vi "Initialize.vi"(7 "Serial Configuration":T1={"Baud Rate"=57600, "Parity"=1, "Data Bits"=7, "Stop Bits"=10, "Flow Control"=0} {"Flow Control" items=["None", "XON/XOFF", "RTS/CTS", "XON/XOFF & RTS/CTS", "DTR/DSR", "XON/XOFF & DTR/DSR"]; "Stop Bits" items=["1.0"=10, "1.5"=15, "2.0"=20]; "Data Bits" items=["7"=7, "8"=8]; "Parity" items=["None", "Odd", "Even", "Mark", "Space"]; "Baud Rate" items=["300"=300, "600"=600, "1200"=1200, "2400"=2400, "4800"=4800, "9600"=9600, "19200"=19200, "38400"=38400, "57600"=57600]}, 8 "error in (no error)":errorcluster, 9 "Reset (True)":bool=TRUE, 10 "ID Query (True)":bool=TRUE, 11 "VISA resource name":refnum<visa-resource-name>) -> (0 "error out":errorcluster, 3 "VISA resource name out":refnum<visa-resource-name>)   [LabVIEW 2015, in "Lake Shore 350.lvlib"]
doc: "Establishes communication with the instrument and optionally performs an instrument identification query and/or an instrument reset. It also places the instrument in a default state needed for other instrument driver operations. Therefore, call this VI before calling other instrument driver VIs for this instrument. Generally, you need to call the <B>Initialize VI</B> only once at the beginning of an application."
uses:
  Lake Shore 350.lvlib
panel:
  # "(c) 2013 Lake Shore Cryotronics Inc.  ALL RIGHTS RESERVED."
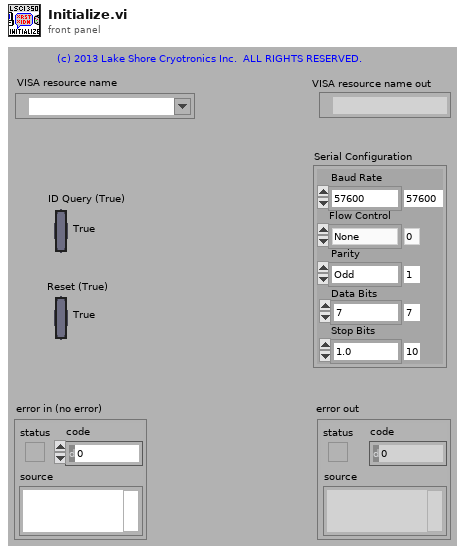
[diagram p1: front panel]
types:
  T1 = cluster{"Baud Rate":u32, "Parity":u16, "Data Bits":u16, "Stop Bits":u16, "Flow Control":u16}
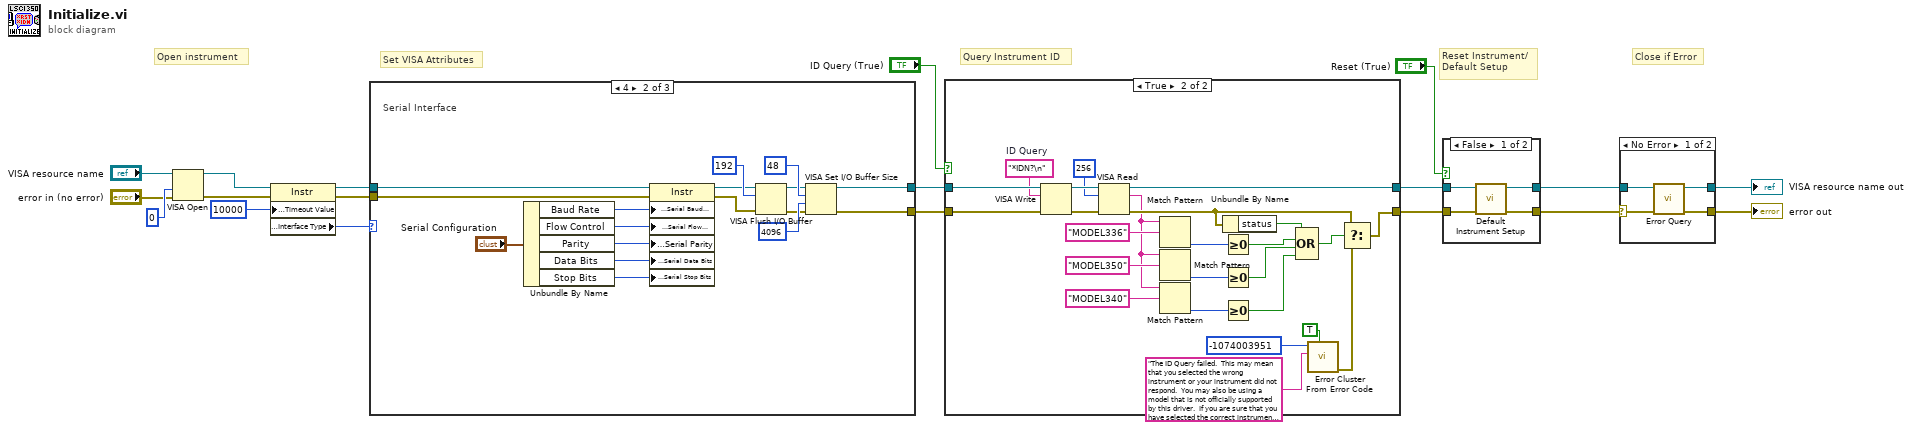
[diagram p0: block diagram]
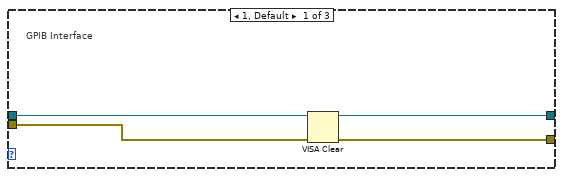
[diagram p2: hidden frame]
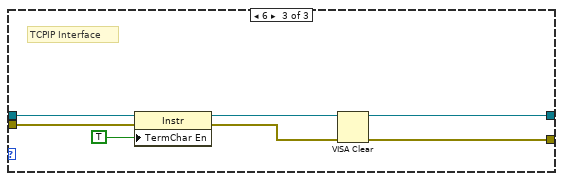
[diagram p3: hidden frame]
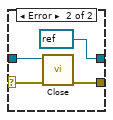
[diagram p4: hidden frame]
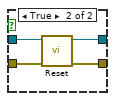
[diagram p5: hidden frame]
diagram:
  # "Set VISA Attributes"
  # "Close if Error"
  # "Query Instrument ID"
  # "Reset Instrument/\nDefault Setup"
  # "Open instrument"
  n1 = VISA Open(access mode=u32 0, error in (no error)="error in (no error)", VISA resource name="VISA resource name") -> (VISA resource name=w9:refnum<visa-resource-name>, error out=w8:errorcluster)  [unwired: 2 in]
  n2 = property class="Instr"(reference=w9, error in=w8, "General Settings:Timeout Value"=u32 10000) -> (reference out=w7:refnum<visa-resource-name>, error out=w6:errorcluster, "Interface Information:Interface Type"=w5:u16)
  n3 = case shown="4" w5 {
    tunnel: [w23 w27 w43] -> w2
    tunnel: [w22 w26 w41] -> w1
    tunnel: w7 -> [w20 w24 w47]
    tunnel: w6 -> [w21 w25 w46]
    frame 1, Default {
      # "GPIB Interface"
      n4 = VISA Clear(VISA resource name=w20, error in (no error)=w21) -> (VISA resource name out=w23:refnum<visa-resource-name>, error out=w22:errorcluster)
    }
    frame 4 {
      # "Serial Interface"
      n5 = Unbundle By Name("Serial Configuration") -> ("Baud Rate"=w35:u32, "Flow Control"=w39:u16, "Parity"=w37:u16, "Data Bits"=w36:u16, "Stop Bits"=w40:u16)
      n6 = property class="Instr"(reference=w24, error in=w25, "Serial Settings:Serial Baud Rate"=w35, "Serial Settings:Serial Flow Control"=w39, "Serial Settings:Serial Parity"=w37, "Serial Settings:Serial Data Bits"=w36, "Serial Settings:Serial Stop Bits"=w40) -> (reference out=w31:refnum<visa-resource-name>, error out=w29:errorcluster)
      n7 = VISA Flush I/O Buffer(VISA resource name=w31, mask (16)=u16 192, error in (no error)=w29) -> (VISA resource name out=w28:refnum<visa-resource-name>, error out=w30:errorcluster)
      n8 = VISA Set I/O Buffer Size(VISA resource name=w28, mask (16)=u16 48, size (4096)=u32 4096 ("size (0)"), error in (no error)=w30) -> (VISA resource name out=w27:refnum<visa-resource-name>, error out=w26:errorcluster)
    }
    frame 6 {
      # "TCPIP Interface"
      n9 = property class="Instr"(reference=w47, error in=w46, "TermChar En"=TRUE) -> (reference out=w44:refnum<visa-resource-name>, error out=w42:errorcluster)
      n10 = VISA Clear(VISA resource name=w44, error in (no error)=w42) -> (VISA resource name out=w43:refnum<visa-resource-name>, error out=w41:errorcluster)
    }
  }
  n11 = case shown="True" "ID Query (True)" {
    tunnel: [w48 w74] -> w18
    tunnel: [w49 w59] -> w19
    tunnel: w2 -> [w49 w72]
    tunnel: w1 -> [w48 w73]
    frame False {
    }
    frame True {
      w60 = "*IDN?\n"  # ID Query
      n12 = VISA Write(VISA resource name=w72, write buffer=w60, error in (no error)=w73) -> (VISA resource name out=w71:refnum<visa-resource-name>, error out=w70:errorcluster)  [unwired: 1 out]
      n13 = VISA Read(VISA resource name=w71, byte count=u32 256, error in (no error)=w70) -> (VISA resource name out=w59:refnum<visa-resource-name>, read buffer=w50:string, error out=w58:errorcluster)  [unwired: 1 out]
      n14 = Match Pattern(string=w50, regular expression="MODEL336") -> (offset past match=w64:i32)  [unwired: 1 in, 3 out]
      n15 = Match Pattern(string=w50, regular expression="MODEL350") -> (offset past match=w55:i32)  [unwired: 1 in, 3 out]
      n16 = Match Pattern(string=w50, regular expression="MODEL340") -> (offset past match=w53:i32)  [unwired: 1 in, 3 out]
      n17 = Unbundle By Name(w58) -> ("status"=w63:bool)
      n18 = Greater Or Equal To 0?(x=w64) -> (x >= 0?=w61:bool)
      n19 = Greater Or Equal To 0?(x=w55) -> (x >= 0?=w54:bool)
      n20 = Greater Or Equal To 0?(x=w53) -> (x >= 0?=w51:bool)
      n21 = Compound Arithmetic op=OR(w63, w61, w54, w51) -> (w62:bool)
      n22 = call <vilib>:"Error Cluster From Error Code.vi"("show call chain? (False)"=TRUE, "error message (\"\")"="The ID Query failed.  This may mean that you selected the wrong instrument or your instrument did not respond.  You may also be using a model that is not officially supported by this driver.  If you are sure that you have selected the correct instrument and it is responding, try disabling the ID Query." ("Source (VI Name)"), "error code (0)"=-1074003951 ("Code")) -> ("error out"=w68:errorcluster)  [unwired: 6 in]
      n23 = Select(t=w58, s=w62, f=w68) -> (s? t:f=w74:errorcluster)
    }
  }
  n24 = case shown="False" "Reset (True)" {
    tunnel: w18 -> [w77 w79]
    tunnel: [w76 w82] -> w12
    tunnel: w19 -> [w78 w80]
    tunnel: [w75 w81] -> w13
    frame False {
      n25 = call "Default Instrument Setup.vi"("error in (no error)"=w77, "VISA resource name"=w78) -> ("error out"=w76:errorcluster, "VISA resource name out"=w75:refnum<visa-resource-name>)  [unwired: 8 in]
    }
    frame True {
      n26 = call "Reset.vi"("error in (no error)"=w79, "VISA resource name"=w80) -> ("error out"=w82:errorcluster, "VISA resource name out"=w81:refnum<visa-resource-name>)  [unwired: 8 in]
    }
  }
  n27 = case shown="No Error" w12 {
    selector: w12 -> [w86 w88]
    tunnel: w13 -> [w85 w89]
    tunnel: [w84 refnum<visa-resource-name> refnum ("VISA resource name out")] -> w15
    tunnel: [w83 w90] -> w14
    frame No Error {
      n28 = call "Error Query.vi"("error in (no error)"=w86, "VISA resource name"=w85) -> ("error out"=w83:errorcluster, "VISA resource name out"=w84:refnum<visa-resource-name>)  [unwired: 7 in, 1 out]
    }
    frame Error {
      n29 = call "Close.vi"("error in (no error)"=w88, "VISA resource name"=w89) -> ("error out"=w90:errorcluster)  [unwired: 9 in]
    }
  }
  "VISA resource name out" <- w15
  "error out" <- w14
